vi "Walk Path.vi"(7 "Next Node Map":T1(c390), 8 "End":cluster{"Row":i32, "Col":i32}, 10 "Distance In":i64, 11 "Path In":cluster{"Row":i32, "Col":i32}[](array[cluster])) -> (2 "Distance Out":i64)   [LabVIEW 2021]
uses:
  ddac44cb-6b46-4377-8674-6b0f2d57a36d.vi
  <vilib>/Comparison/Equal/Equal Functor/Equal Functor.lvclass
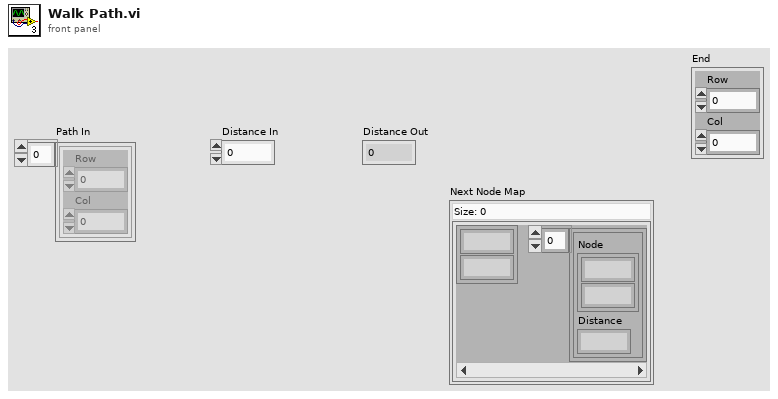
[diagram p1: front panel]
types:
  T1 = map{cluster{i32, i32}, cluster{"Node":cluster{i32, i32}, "Distance":i64}[]}
  T2 = cluster{"Node":cluster{i32, i32}, "Distance":i64}[]
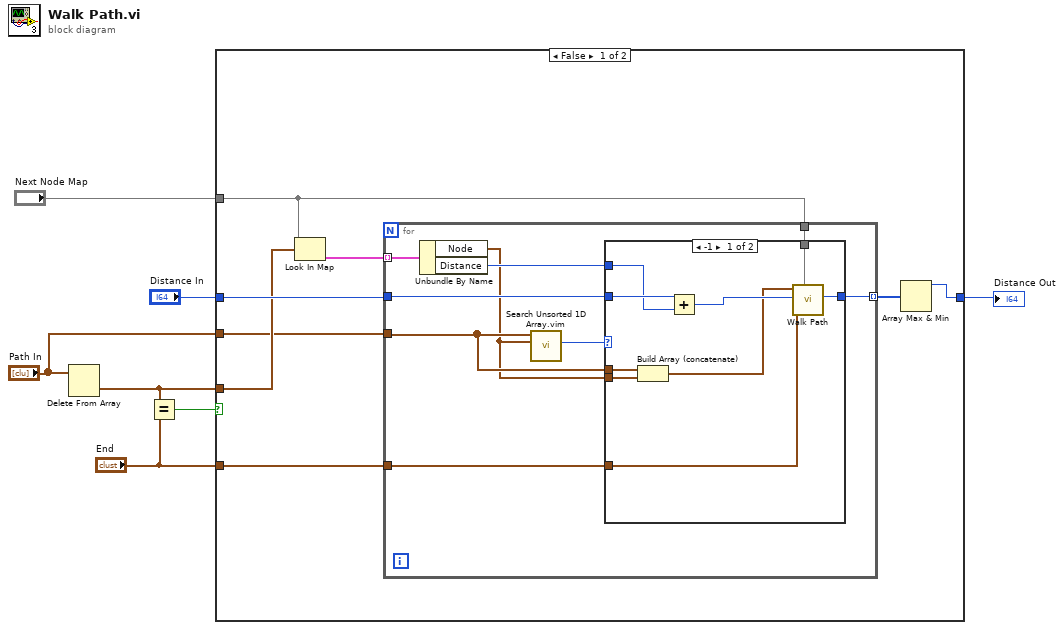
[diagram p0: block diagram]
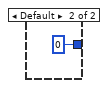
[diagram p2: hidden frame]
diagram:
  n1 = Delete From Array(array="Path In") -> (deleted portion=w2:cluster{"Row":i32, "Col":i32})  [unwired: 2 in, 1 out]
  n2 = Equal?(x=w2, y="End") -> (x = y?=w7:bool)
  n3 = case shown="False" w7 {
    tunnel: "Distance In" -> [w13 w35]
    tunnel: [w12 w35] -> w5
    tunnel: "End" -> [w15 _]
    tunnel: "Next Node Map" -> [w8 _]
    tunnel: w2 -> [w11 _]
    tunnel: "Path In" -> [w9 _]
    frame False {
      n4 = Look In Map(map=w8, key=w11) -> (value=w10:T2)  [unwired: 1 in, 1 out]
      n5 = for {
        tunnel: w15 -> [w24]
        tunnel: w13 -> [w22]
        tunnel: [w23] -> w14 mode=indexing
        tunnel: w10 -> [w21] mode=indexing
        tunnel: w9 -> [w18]
        tunnel: w8 -> [w16]
        n6 = Unbundle By Name(w21) -> ("Node"=w17:cluster{i32, i32}, "Distance"=w19:i64)
        n7 = call "Search Unsorted 1D Array.vim"("element"=w17, "unsorted 1D array"=w18) -> ("index of element"=w20:i32)  [unwired: 9 in]
        n8 = case shown="-1" w20 {
          tunnel: w24 -> [w33 _]
          tunnel: [w32 i64 0 ("Distance Out")] -> w23
          tunnel: w22 -> [w30 _]
          tunnel: w19 -> [w29 _]
          tunnel: w18 -> [w28 _]
          tunnel: w17 -> [w27 _]
          tunnel: w16 -> [w25 _]
          frame -1 {
            n9 = Build Array (concatenate)(w28, w27) -> (w26:cluster{"Row":i32, "Col":i32}[])
            n10 = Add(x=w30, y=w29) -> (x+y=w31:i64)
            n11 = call "Walk Path.vi"("Next Node Map"=w25, "End"=w33, "Distance In"=w31, "Path In"=w26) -> ("Distance Out"=w32:i64)  [unwired: 7 in]
          }
          frame Default {
          }
        }
      }
      n12 = Array Max & Min(array=w14) -> (max value=w12:i64)  [unwired: 3 out]
    }
    frame True {
    }
  }
  "Distance Out" <- w5
